vi "SVT UFF58 Write Spectrum (Real) (1 Ch).vi"(0 "file refnum":refnum<k20>, 1 "ID lines (1-3)":T8, 2 "data precision (double-precision:1)":T1=1 items=["single-precision", "double-precision"], 5 "spectrum":cluster{"x0":dbl, "dx":dbl, "Y":dbl[]} {"Y" format="%.2p"; "dx" format="%.2p"; "x0" format="%.2p"}, 9 "spectrum info":T2={"channel name"="", "description"="", "x-axis units"=0, "spectral info"={"spectrum type"=enum."Power [Magnitude^2]", "linear/dB"=enum."linear", "window"=0, "window size"=0, "FFT size"=0}, "engineering units"=0, "custom label"="", "dB reference [EU]"=0.0, "peak units"=enum."rms", "weighting filter"=0, "spectral density?"=FALSE, "unit label"="", "spectrum skewed?"=FALSE, "complimentary spectrum units"=enum."none"} {"x-axis units" items=["Time (s)"=0, "Frequency-CB (Hz)"=1, "Frequency-CPB (Hz)"=1248, "Frequency-Arbitrary (Hz)"=2357, "Quefrency (s)"=2, "Revolutions (rev)"=3, "Order"=4, "Speed (RPM)"=11, "Speed (rad/s)"=21, "Index"=65535]; "weighting filter" items=["Linear", "A-weighting", "B-weighting", "C-weighting", "ITU-R 468-4", "Dolby", "CCITT", "C-message", "Wb", "Wc", "Wd", "We", "Wf", "Wh", "Wj", "Wk", "Wm", "AES17 20 kHz lowpass", "AES17 40 kHz lowpass", "AES17 20 kHz highpass", "AES17 40 kHz highpass"]; "dB reference [EU]" format="%.2f"; "engineering units" items=["custom..."=0, "V"=1, "A"=21, "C"=30, "pC"=31, "s"=32, "-"=29, "Pa"=2, "N"=20, "g"=3, "m/s^2"=4, "m/s"=5, "m"=6, "mm/s"=12, "mm"=13, "micron/s"=14, "micron"=15, "in/s^2"=7, "in/s"=8, "in"=9, "mil/s"=10, "mil"=11, "rad/s^2"=16, "rad/s"=17, "rad"=18, "deg/s^2"=26, "deg/s"=27, "deg"=28, "RPM"=22, "cycle/s^2"=23, "Hz"=24, "cycle"=25, "strain"=19]; "spectral info"."window" items=["None "=0, "Hanning"=1, "Hamming"=2, "Blackman-Harris"=3, "Exact Blackman"=4, "Blackman"=5, "Flat Top"=6, "4 Term B-Harris "=7, "7 Term B-Harris"=8, "Low Sidelobe"=9, "Force - Exponential"=10, "Gaussian"=62]}, 11 "error in (no error)":errorcluster) -> (4 "dup file refnum":refnum<k20>, 6 "function refnum":refnum<k20>, 15 "error out":errorcluster)   [LabVIEW 2017, in "SoundVib_UFF58.lvlib"]
doc: "Writes data to the UFF58 (universal file format) file specified by the <B>file refnum</B> input. This VI also writes the fields in records 1, 2, and 3, <B>ID lines (1-3)</B>. You can write a single time domain waveform, multiple time domain waveforms, a single real frequency spectrum, multiple real frequency spectra, a single complex frequency spectrum, multiple complex frequency spectra, or generic data to a UFF file. If a frequency spectrum is in decibels, this VI converts the spectrum to linear before writing to the UFF58 file. The default instance, SVT UFF58 Write Time Waveform (1 Ch), writes a single time domain waveform to the file specified by the <B>file refnum</B> input. Wire data to the <B>file refnum</B> input to determine the polymorphic instance to use or manually select the instance."
uses:
  <vilib>/addons/Sound and Vibration/svt_UFF58/SoundVib_UFF58.lvlib
  <vilib>/addons/Sound and Vibration/svt_UFF58/subVIs/sv_IDLines123.ctl
  <vilib>/addons/_NISVFA/_Shared subVIs/Controls/svc_Spectrum Info.ctl
  <vilib>/addons/_NISVFA/_Shared subVIs/Controls/svc_X-Axis Units.ctl
  <vilib>/addons/_NISVFA/_Shared subVIs/Controls/svc_Spectrum Type.ctl
  <vilib>/addons/_NISVFA/_Shared subVIs/Controls/svc_Engineering Units Text Ring.ctl
  <vilib>/addons/_NISVFA/_Shared subVIs/Controls/svc_Weighting Filter Text Ring.ctl
  <vilib>/addons/_NISVFA/_Shared subVIs/Controls/svc_Complimentary Spectrum Units.ctl
  <vilib>/addons/Sound and Vibration/svt_UFF58/subVIs/sv_UFF58 Data Precision.ctl
  <vilib>/addons/Sound and Vibration/svt_UFF58/subVIs/sv_UFF58 Check Data Valid (Freq - Real) (1Ch).vi
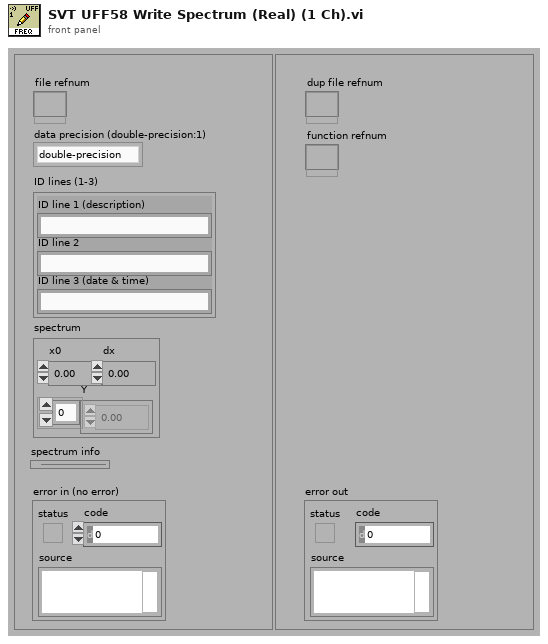
[diagram p1: front panel]
types:
  T1 = typedef "SoundVib_UFF58.lvlib/sv_UFF58 Data Precision.ctl" = u32
  T2 = typedef "svc_Spectrum Info.ctl" = cluster{"channel name":string, "description":string, "x-axis units":T3, "spectral info":cluster{"spectrum type":T4, "linear/dB":enum16{"linear", "dB"}, "window":u16, "window size":i32, "FFT size":i32}, "engineering units":T5, "custom label":string, "dB reference [EU]":dbl, "peak units":enum16{"rms", "peak", "peak-peak"}, "weighting filter":T6, "spectral density?":bool, "unit label":string, "spectrum skewed?":bool, "complimentary spectrum units":T7}
  T3 = typedef "svc_X-Axis Units.ctl" = u16
  T4 = typedef "svc_Spectrum Type.ctl" = enum16{"FFT Spectrum [complex]", "Amplitude [Magnitude]", "Power [Magnitude^2]", "Cross Spectrum [complex]", "Frequency Response [Complex]"}
  T5 = typedef "svc_Engineering Units Text Ring.ctl" = u16
  T6 = typedef "svc_Weighting Filter Text Ring.ctl" = u16
  T7 = typedef "svc_Complimentary Spectrum Units.ctl" = enum16{"none", "radians", "degrees", "cycles", "imaginary"}
  T8 = typedef "SoundVib_UFF58.lvlib/sv_IDLines123.ctl" = cluster{"ID line 1 (description)":string, "ID line 2":string, "ID line 3 (date & time)":string}
  T9 = typedef "SoundVib_UFF58.lvlib/sv_UFF58 DOF.ctl" = cluster{"function type":T10, "function ID number":i32, "version number":i32, "load case ID number":i32, "response entity name":string, "response node":i32, "response direction":T11, "reference entity name":string, "reference node":i32, "reference direction":T11}
  T10 = typedef "SoundVib_UFF58.lvlib/sv_FunctionType.ctl" = enum16{"general or unknown", "time response", "auto spectrum", "cross spectrum", "frequency response function", "transmissibility", "coherence", "auto correlation", "cross correlation", "power spectral density (PSD)", "energy spectral density (ESD)", "probability density function", "spectrum", "cumulative frequency distribution", "peaks valley", "stress/cycles", "strain/cycles", "orbit", "mode indicator function", "force pattern", "partial power", "partial coherence", "eigenvalue", "eigenvector", "shock response spectrum", "finite impulse response filter", "multiple coherence", "order function", "phase compensation"}
  T11 = typedef "SoundVib_UFF58.lvlib/sv_UFF58 Response Direction.ctl" = i32
  T12 = typedef "SoundVib_UFF58.lvlib/sv_UFF58 Axis Characteristics.ctl" = cluster{"specific data type":T13, "length units exponent":i32, "force units exponent":i32, "temperature units exponent":i32, "axis label":string, "axis units label":string}
  T13 = typedef "SoundVib_UFF58.lvlib/sv_UFF58 Specific Datatype.ctl" = u16
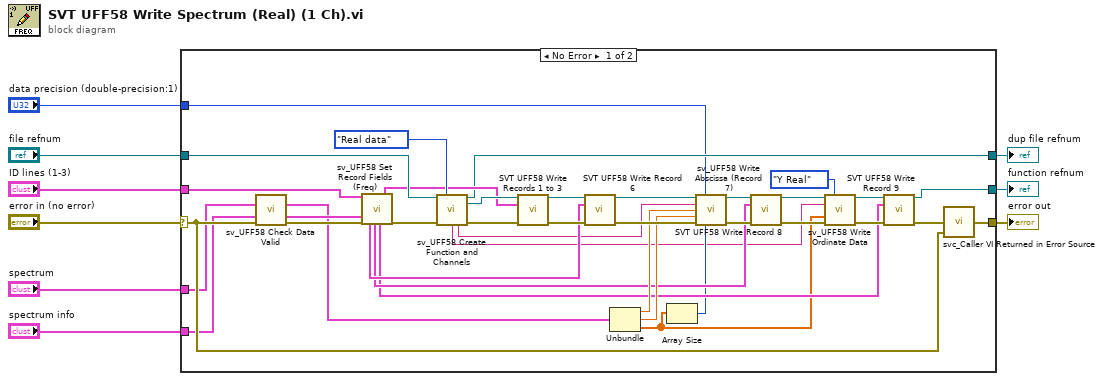
[diagram p0: block diagram]
diagram:
  n1 = case shown="No Error" "error in (no error)" {
    selector: "error in (no error)" -> [w20 w48]
    tunnel: [w21 w48] -> w9
    tunnel: "ID lines (1-3)" -> [w43 _]
    tunnel: [w17 w49] -> w7
    tunnel: "file refnum" -> [w37 w49]
    tunnel: "spectrum" -> [w19 _]
    tunnel: "spectrum info" -> [w13 _]
    tunnel: [w31 _] -> w2
    tunnel: "data precision (double-precision:1)" -> [w14 _]
    frame No Error {
      n2 = call-poly <vilib>:"sv_UFF58 Check Data Valid.vi"("spectrum in"=w19, "spectrum info"=w13, "error in (no error)"=w20) -> ("spectrum out"=w11:cluster{"f0":dbl, "df":dbl, "magnitude":dbl[]}, "spectrum info out"=w12:T2, "error out"=w46:errorcluster)  [unwired: 10 in]
      n3 = call <vilib>:"sv_UFF58 Set Record Fields (Freq).vi"("ID lines (1-3)"=w43, "spectrum info"=w12, "error in (no error)"=w46) -> ("DOF identification (record 6)"=w40:T9, "abscissa data characteristics (record 8)"=w27:T12, "ordinate numerator data characteristics (record 9)"=w26:T12, "ID lines (1-3) out"=w18:T8, "error out"=w28:errorcluster)  [unwired: 11 in, 1 out]
      n4 = call <vilib>:"sv_UFF58 Create Function and Channels.vi"("file refnum"=w37, "real or complex data?"=enum16{"Real data", "Complex data"}."Real data", "error in (no error)"=w28) -> ("dup file refnum"=w17:refnum<k20>, "function refnum"=w36:refnum<k20>, "ordinate numerator channel name"=w15:string, "abscissa channel name"=w16:string, "error out"=w35:errorcluster)  [unwired: 6 in, 2 out]
      n5 = call <vilib>:"SVT UFF58 Write Records 1 to 3.vi"("function refnum"=w36, "ID lines (1-3)"=w18, "error in (no error)"=w35) -> ("dup function refnum"=w42:refnum<k20>, "error out"=w41:errorcluster)  [unwired: 11 in]
      n6 = call <vilib>:"SVT UFF58 Write Record 6.vi"("function refnum"=w42, "DOF identification"=w40, "error in (no error)"=w41) -> ("dup function refnum"=w30:refnum<k20>, "error out"=w47:errorcluster)  [unwired: 11 in]
      n7 = Unbundle(w11) -> ("f0"=w44:dbl, "df"=w45:dbl, "magnitude"=w24:dbl[])
      n8 = Array Size(array=w24) -> (size(s)=w23:i32)
      n9 = call <vilib>:"sv_UFF58 Write Abscissa (Record 7).vi"("function refnum"=w30, "data precision (double-precision:1)"=w14, "Name"=w16, "x0"=w44, "dx"=w45, "error in (no error)"=w47, "channel length"=w23) -> ("dup function refnum"=w39:refnum<k20>, "error out"=w38:errorcluster)  [unwired: 7 in]
      n10 = call <vilib>:"SVT UFF58 Write Record 8.vi"("function refnum"=w39, "abscissa data characteristics"=w27, "error in (no error)"=w38) -> ("dup function refnum"=w29:refnum<k20>, "error out"=w33:errorcluster)  [unwired: 11 in]
      n11 = call <vilib>:"sv_UFF58 Write Ordinate Data.vi"("function refnum"=w29, "channel to write"=enum16{"X", "Y Real", "Y Imaginary"}."Y Real", "ordinate channel name"=w15, "ordinate data"=w24, "error in (no error)"=w33) -> ("dup function refnum"=w32:refnum<k20>, "error out"=w34:errorcluster)  [unwired: 9 in]
      n12 = call <vilib>:"SVT UFF58 Write Record 9.vi"("function refnum"=w32, "ordinate data characteristics"=w26, "error in (no error)"=w34) -> ("dup function refnum"=w31:refnum<k20>, "error out"=w10:errorcluster)  [unwired: 11 in]
      n13 = call <vilib>:"svc_Caller VI Returned in Error Source.vi"("warning input to caller"=w20, "error in (no error)"=w10) -> ("error out"=w21:errorcluster)  [unwired: 3 in]
    }
    frame Error {
    }
  }
  "dup file refnum" <- w7
  "error out" <- w9
  "function refnum" <- w2
